vi "Default.File.MD5Checksum Files.vi"(8 "error in (no error)":errorcluster, 11 "FilePaths":path[](array[path])) -> (0 "error out":errorcluster, 2 "Checksum Array":string[](array[string]), 3 "MD5 message-digest":string)   [LabVIEW 2010]
doc: "Create an MD5 message-digest for a list of files."
uses:
  MD5 Message Digest (Hexadecimal String)__ogtk.vi
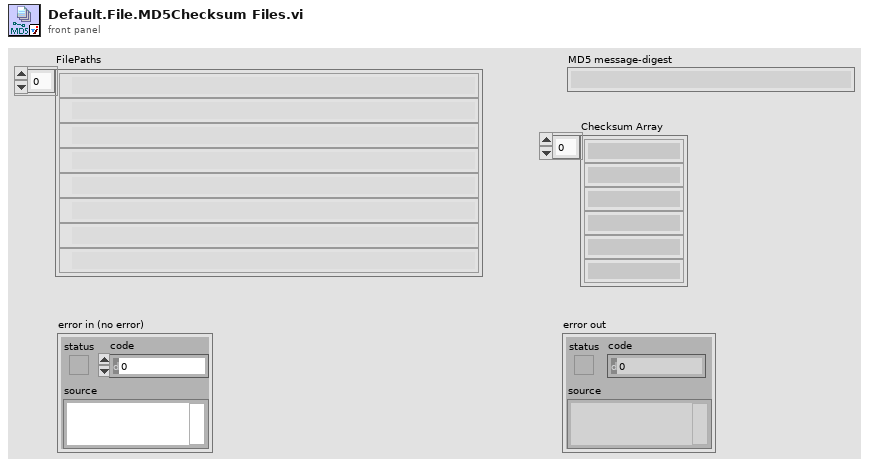
[diagram p1: front panel]
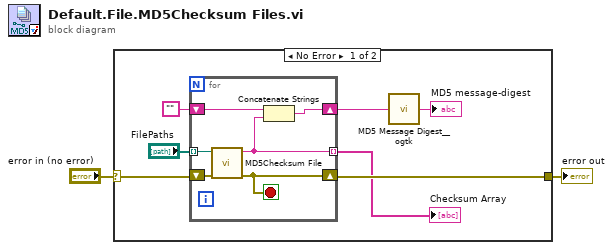
[diagram p0: block diagram]
diagram:
  n1 = case shown="No Error" "error in (no error)" {
    selector: "error in (no error)" -> [w5 w16]
    tunnel: [w8 w16] -> w1
    frame No Error {
      n2 = for {
        shift-right: [w11] -> w8
        shift-left: w5 -> [w14]
        tunnel: "FilePaths" -> [w15] mode=indexing
        shift-right: [w12] -> w7
        shift-left: "" -> [w13]
        tunnel: [w10] -> w3 mode=indexing
        stop <- w11 stop-if-true
        n3 = call <vilib>:"MD5Checksum File.vi"("error in (no error)"=w14, "Path"=w15) -> ("error out"=w11:errorcluster, "MD5 message-digest"=w10:string)  [unwired: 8 in]
        n4 = Concatenate Strings(w13, w10) -> (w12:string)
      }
      "Checksum Array" <- w3
      n5 = call-poly "MD5 Message Digest__ogtk.vi"("Message"=w7) -> ("MD5 Message Digest"=→"MD5 message-digest":string)
    }
    frame Error {
    }
  }
  "error out" <- w1
